vi "test-bang-bang-input-output.vi"(8 "error in (no error)":errorcluster) -> (0 "error out":errorcluster, 3 "All Tests Passed":bool)   [LabVIEW 2019]
uses:
  <vilib>/Rock Robotics/WPI/ThirdParty/JAS_Junk/TrajLib/BangBang_SetTolerance.vi
  <vilib>/Rock Robotics/WPI/ThirdParty/JAS_Junk/TrajLib/Trajectory_Library.lvlib
panel:
  out "Test Passed 1":bool
  out "Test Passed 0":bool
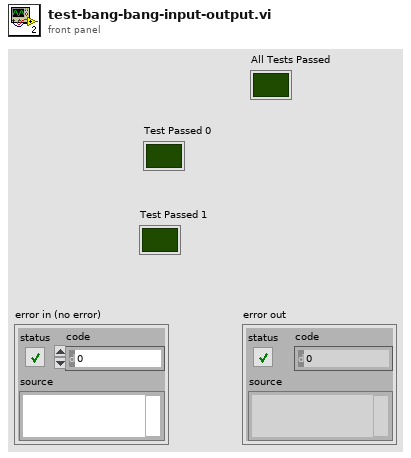
[diagram p1: front panel]
types:
  T1 = typedef "Trajectory_Library.lvlib/BANG_BANG.ctl" = cluster{"Tolerance":dbl, "Setpoint":dbl, "Measurment":dbl}
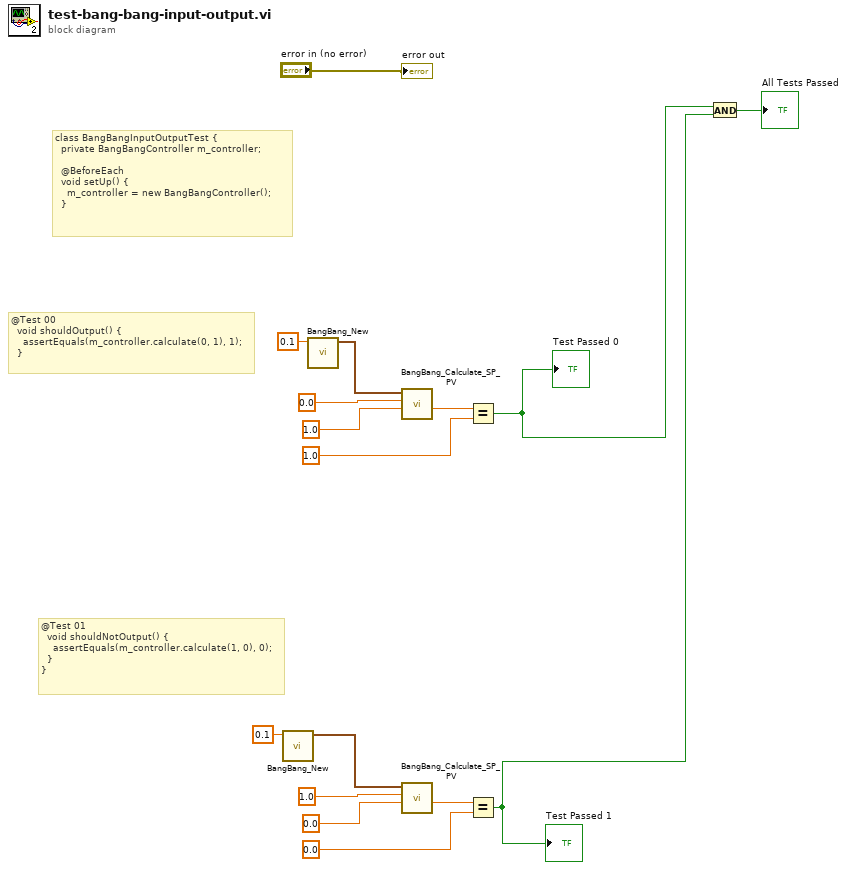
[diagram p0: block diagram]
diagram:
  # "@Test 01\n  void shouldNotOutput() {\n    assertEquals(m_controller.calculate(1, 0), 0);\n  }\n}"
  # "@Test 00\n  void shouldOutput() {\n    assertEquals(m_controller.calculate(0, 1), 1);\n  }"
  # "class BangBangInputOutputTest {\n  private BangBangController m_controller;\n\n  @BeforeEach\n  void setUp() {\n    m_controller = new BangBangController();\n  }"
  n1 = call <vilib>:"BangBang_New.vi"("Tolerance"=0.1) -> ("BANG_BANG"=w6:T1)  [unwired: 10 in]
  n2 = call <vilib>:"BangBang_New.vi"("Tolerance"=0.1) -> ("BANG_BANG"=w13:T1)  [unwired: 10 in]
  n3 = call <vilib>:"BangBang_Calculate_SP_PV.vi"("Setpoint"=1.0, "Measurment"=0.0, "BANG_BANG"=w13) -> ("ControlOutput"=w10:dbl)  [unwired: 7 in, 1 out]
  n4 = call <vilib>:"BangBang_Calculate_SP_PV.vi"("Setpoint"=0.0, "Measurment"=1.0, "BANG_BANG"=w6) -> ("ControlOutput"=w3:dbl)  [unwired: 7 in, 1 out]
  n5 = Equal?(x=w10, y=1.0) -> (x = y?=w8:bool)
  "Test Passed 0" <- w8
  n6 = Equal?(x=w3, y=0.0) -> (x = y?=w1:bool)
  "Test Passed 1" <- w1
  n7 = And(x=w8, y=w1) -> (x .and. y?=→"All Tests Passed":bool)
  "error out" <- "error in (no error)"
